vi "daq.vi"(2 "Control Array":dbl[](array[numeric]), 3 "DAQ?":bool, 4 "Parametros Interferometro/DAQ":T2, 5 "#samples":u32, 7 "DAQ Device IN":T1={"DAQ Fs (S/s)"=10000.0, "task"="", "error"={"status"=FALSE, "code"=0, "source"=""}}) -> (0 "Waveform":waveform(dbl), 1 "DAQ Device OUT":T1)   [LabVIEW 2010]
uses:
  <vilib>/DAQmx/write.llb/DAQmx Write (Analog Wfm 1Chan NSamp).vi
  <vilib>/daqmx/miscellaneous.llb/DAQmx Fill In Error Info.vi
panel:
  out "Waveform Graph":waveform(dbl)(graph)
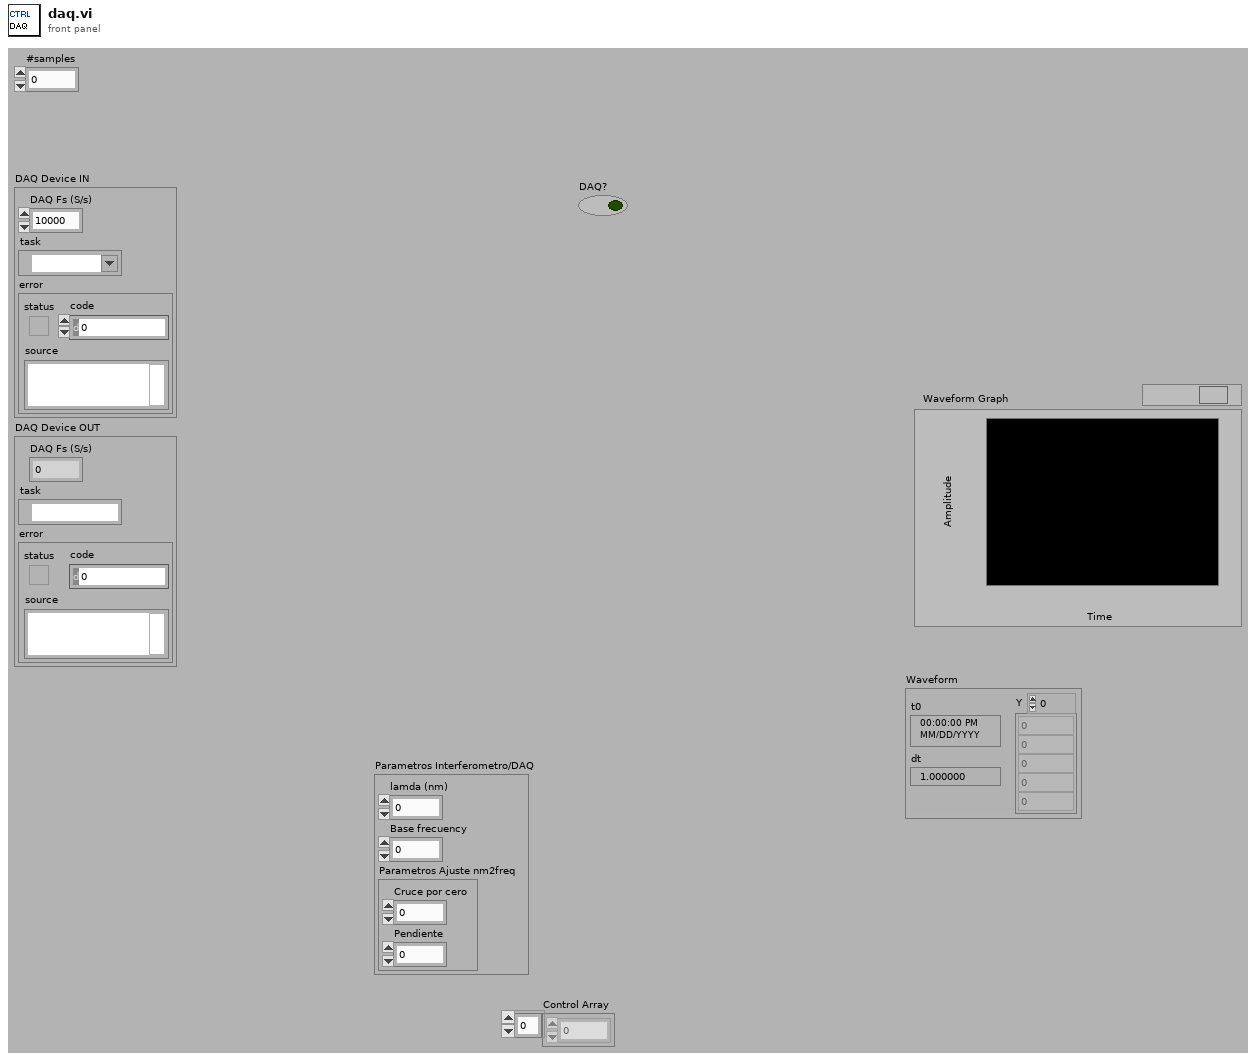
[diagram p1: front panel]
types:
  T1 = cluster{"DAQ Fs (S/s)":dbl, "task":refnum<k21>, "error":errorcluster}
  T2 = cluster{"lamda (nm)":dbl, "Base frecuency":dbl, "Parametros Ajuste nm2freq":cluster{"Cruce por cero":dbl, "Pendiente":dbl}}
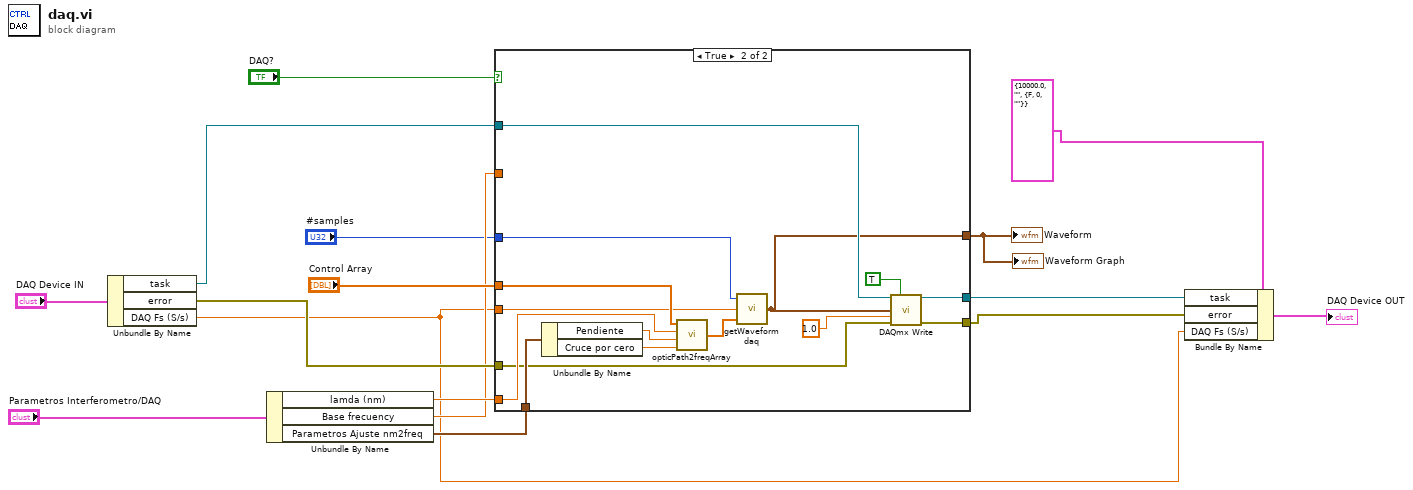
[diagram p0: block diagram]
diagram:
  n1 = Unbundle By Name("DAQ Device IN") -> ("task"=w14:refnum<k21>, "error"=w13:errorcluster, "DAQ Fs (S/s)"=w4:dbl)
  n2 = Unbundle By Name("Parametros Interferometro/DAQ") -> ("lamda (nm)"=w10:dbl, "Base frecuency"=w9:dbl, "Parametros Ajuste nm2freq"=w8:cluster{"Cruce por cero":dbl, "Pendiente":dbl})
  n3 = case shown="True" "DAQ?" {
    tunnel: w14 -> [w17 w25]
    tunnel: [w17 w26] -> w3
    tunnel: w13 -> [w18 w23]
    tunnel: [w18 w24] -> w12
    tunnel: w4 -> [_ w27]
    tunnel: w9 -> [_ _]
    tunnel: "Control Array" -> [_ w31]
    tunnel: "#samples" -> [_ w19]
    tunnel: w10 -> [_ w33]
    tunnel: w8 -> [_ w32]
    tunnel: [_ w20] -> w7
    frame False {
    }
    frame True {
      n4 = Unbundle By Name(w32) -> ("Pendiente"=w29:dbl, "Cruce por cero"=w28:dbl)
      n5 = call "opticPath2freqArray.vi"("b"=w28, "m"=w29, "lamda (nm)"=w33, "camino optico (nm)"=w31) -> ("freq"=w30:dbl[])
      n6 = call "getWaveform daq.vi"("df"=w30, "Fs (S/s)"=w27, "#samples"=w19) -> ("Waveform"=w20:waveform(dbl))
      n7 = call-poly <vilib>:"DAQmx Write.vi"("task/channels in"=w25, "auto start"=TRUE, "data"=w20, "timeout"=1.0, "error in"=w23) -> ("task out"=w26:refnum<k21>, "error out"=w24:errorcluster)  [unwired: 8 in, 1 out]
    }
  }
  "Waveform" <- w7
  "Waveform Graph" <- w7
  n8 = Bundle By Name(cluster=T1 {"DAQ Fs (S/s)"=10000.0, "task"="", "error"={"status"=FALSE, "code"=0, "source"=""}} ("DAQ Device"), "task"=w3, "error"=w12, "DAQ Fs (S/s)"=w4) -> (→"DAQ Device OUT":T1)
